vi "graph-real.vi"(8 "error in (no error)":errorcluster, 10 "Sr830 in":refnum<vi>) -> (0 "error out":errorcluster, 2 "Sr830 out":refnum<vi>, 3 "Data":T1)   [LabVIEW 2016]
uses:
  controls/LockIn.ctl
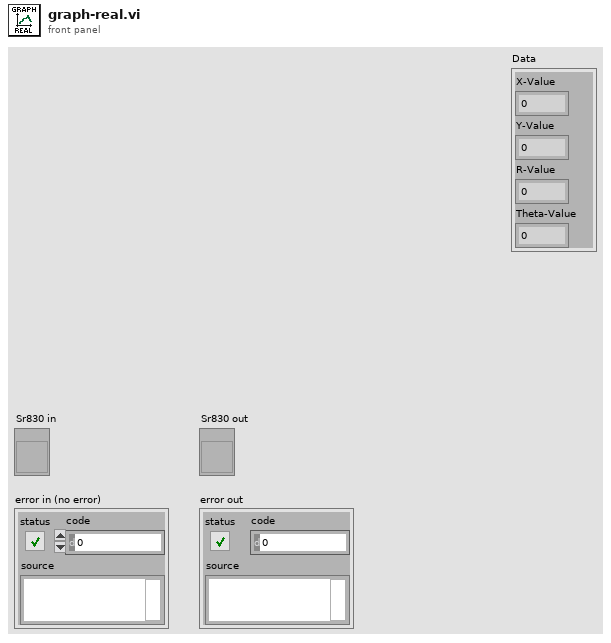
[diagram p1: front panel]
types:
  T1 = cluster{"X-Value":dbl, "Y-Value":dbl, "R-Value":dbl, "Theta-Value":dbl}
  T2 = typedef "LockIn.ctl" = cluster{"Port":refnum<visa-resource-name>, "Is connected?":bool, "Sensivity Ovld":bool, "lockin-open":bool, "lockin-save":bool, "Reference":cluster{"Source ":u16, "Frequency":dbl}, "Channel Display":cluster{"Channel 1":u16, "Channel 2":u16}, "Sensivity":cluster{"Dynamic Reserve":i16, "Sensitivity":i16, "Time Constant":u16, "Low Pass Filter":u16}, "Display":cluster{"Channel One":dbl, "Channel Two":dbl, "Reference":dbl}, "Parameter Values":cluster{"X-Value":dbl, "Y-Value":dbl, "R-Value":dbl, "Theta-Value":dbl, "Aux In 1 Value":dbl, "Aux In 2 Value":dbl, "Aux In 3 Value":dbl, "Aux In 4 Value":dbl, "Reference Frequency":dbl, "Channel 1 Display":dbl, "Channel 2 Display":dbl}}
  T3 = cluster{"X-Value":dbl, "Y-Value":dbl, "R-Value":dbl, "Theta-Value":dbl, "Aux In 1 Value":dbl, "Aux In 2 Value":dbl, "Aux In 3 Value":dbl, "Aux In 4 Value":dbl, "Reference Frequency":dbl, "Channel 1 Display":dbl, "Channel 2 Display":dbl}
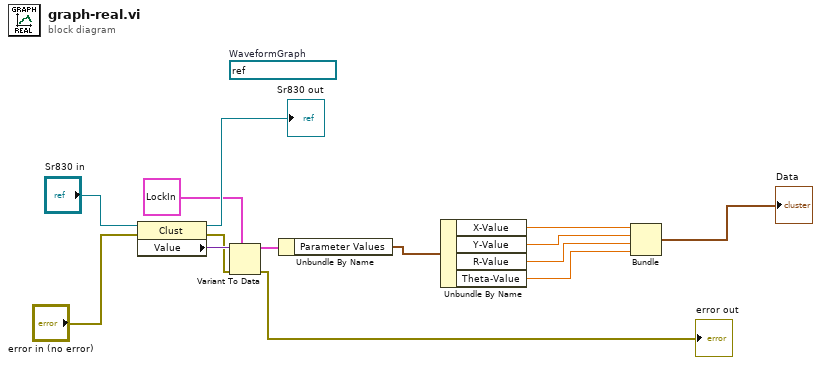
[diagram p0: block diagram]
diagram:
  (unwired) refnum<vi> refnum  # WaveformGraph
  n1 = property class="Clust"(reference="Sr830 in", error in="error in (no error)") -> (reference out=→"Sr830 out":refnum<vi>, error out=w10:errorcluster, "Value"=w11:variant)
  n2 = Variant To Data(error in=w10, type=T2 {"Port"="", "Is connected?"=FALSE, "Sensivity Ovld"=FALSE, "lockin-open"=FALSE, "lockin-save"=FALSE, "Reference"={"Source "=0, "Frequency"=1000.0}, "Channel Display"={"Channel 1"=1, "Channel 2"=1}, "Sensivity"={"Dynamic Reserve"=0, "Sensitivity"=25, "Time Constant"=11, "Low Pass Filter"=2}, "Display"={"Channel One"=0.0, "Channel Two"=0.0, "Reference"=0.0}, "Parameter Values"={"X-Value"=0.0, "Y-Value"=0.0, "R-Value"=0.0, "Theta-Value"=0.0, "Aux In 1 Value"=0.0, "Aux In 2 Value"=0.0, "Aux In 3 Value"=0.0, "Aux In 4 Value"=0.0, "Reference Frequency"=0.0, "Channel 1 Display"=0.0, "Channel 2 Display"=0.0}} ("Lock-In-Amplifier"), Variant=w11) -> (data=w7:T2, error out=→"error out":errorcluster)
  n3 = Unbundle By Name(w7) -> ("Parameter Values"=w2:T3)
  n4 = Unbundle By Name(w2) -> ("X-Value"=w6:dbl, "Y-Value"=w5:dbl, "R-Value"=w4:dbl, "Theta-Value"=w3:dbl)
  n5 = Bundle("X-Value"=w6, "Y-Value"=w5, "R-Value"=w4, "Theta-Value"=w3) -> (→"Data":T1)  [unwired: 1 in]
